vi "Average.vi"(10 "Number 2":dbl, 11 "Number 1":dbl) -> (3 "Average":dbl)   [LabVIEW 2019]
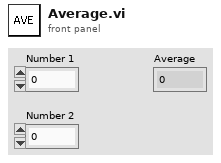
[diagram p1: front panel]
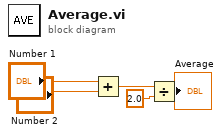
[diagram p0: block diagram]
diagram:
  n1 = Add(x="Number 1", y="Number 2") -> (x+y=w3:dbl)
  n2 = Divide(x=w3, y=2.0) -> (x/y=→"Average":dbl)
